vi "Handle Last Ack Core.vi"(4 "error in (no error)":errorcluster, 6 "Last Ack":refnum<class "Last Ack.lvclass">, 7 "MSS Host Actor in":refnum<class "MSS Host Actor.lvclass">) -> (0 "error out":errorcluster, 3 "MSS Host Actor out":refnum<class "MSS Host Actor.lvclass">)   [LabVIEW 2023, in "MSS Host Actor.lvlib" / "MSS Host Actor.lvclass"]
doc: "(<B>Filename</B>: Actor Framework.lvlib:Actor.lvclass:Handle Last Ack Core.vi)\n\nDefines how the caller actor responds to the Last Ack message from a nested actor. The Last Ack message is the final message a nested actor sends to its caller before it shuts down. The message contains information about the final state of the nested actor.\n\nBy default, this method does nothing except return any error the nested actor sent. A descendant class may override this method to define behavior."
uses:
  MSS Host Actor.lvclass
  <vilib>/ActorFramework/LastAck/Last Ack.lvclass
  Actor-Layers/Mapped Enqueuers/Actor Mapped Enqueuers.lvclass
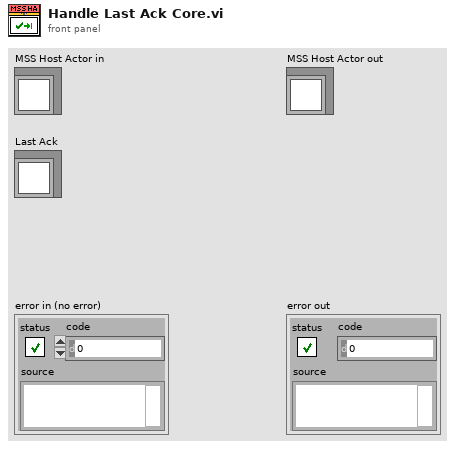
[diagram p1: front panel]
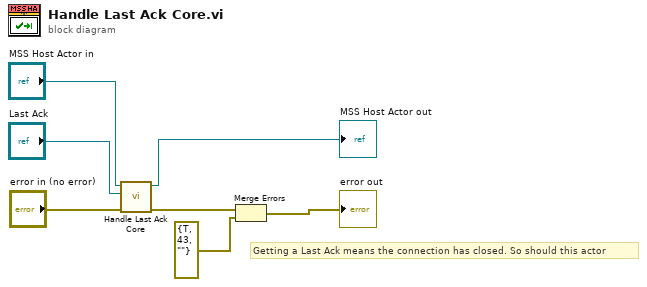
[diagram p0: block diagram]
diagram:
  # "Getting a Last Ack means the connection has closed. So should this actor"
  n1 = call-parent "Handle Last Ack Core.vi"("error in (no error)"="error in (no error)", "Last Ack"="Last Ack", "Actor in"="MSS Host Actor in") -> ("error out"=w7:errorcluster, "Actor out"=→"MSS Host Actor out":refnum<class "MSS Host Actor.lvclass">)  [unwired: 3 in]
  n2 = Merge Errors(w7, errorcluster {"status"=TRUE, "code"=43, "source"=""} ("error in")) -> (→"error out":errorcluster)
